vi "Waveform to XYarray.vi"(1 "Waveform In":waveform(dbl)={"t0"=timestamp(3461330237.7970004 s since 1904-01-01), "dt"=1.0, "Y"=[10.0, 11.3, 9.5]}) -> (0 "Single Plot":cluster{"X array":dbl[], "Y array":dbl[]}={"X array"=[0.0, 1.0, 2.0], "Y array"=[10.0, 11.3, 9.5]})   [LabVIEW 2010]
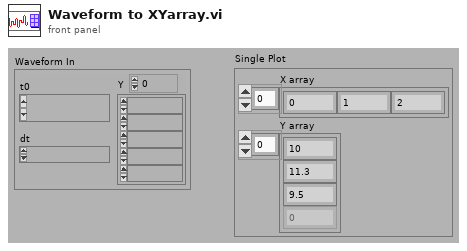
[diagram p1: front panel]
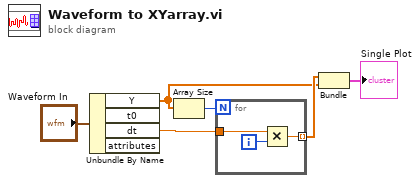
[diagram p0: block diagram]
diagram:
  n1 = Unbundle By Name("Waveform In") -> ("Y"=w1:dbl[], "dt"=w6:dbl)  [unwired: 2 out]
  n2 = Array Size(array=w1) -> (size(s)=w5:i32)
  n3 = for {
    N: w5 -> [_]
    tunnel: w6 -> [w9]
    tunnel: [w8] -> w2 mode=indexing
    i -> [w7]
    n4 = Multiply(x=w9, y=w7) -> (x*y=w8:dbl)
  }
  n5 = Bundle(w2, "Y"=w1) -> (→"Single Plot":cluster{dbl[], "Y":dbl[]})  [unwired: 1 in]
